vi "Set Header.vi"(7 "Replaced Existing (T)":bool=TRUE, 8 "error in (no error)":errorcluster, 9 "Value":string, 10 "Header":string, 11 "Response in":refnum<class "Response.lvclass">) -> (0 "error out":errorcluster, 1 "Replaced":bool, 3 "Response out":refnum<class "Response.lvclass">)   [LabVIEW 2020, in "HTTP Utils.lvlib" / "Response.lvclass"]
uses:
  Response.lvclass
  Response.lvclass/Response.ctl
  <vilib>/Utility/error.llb/Error Cluster From Error Code.vi
  <vilib>/ErrorRing/Error Ring.xnode
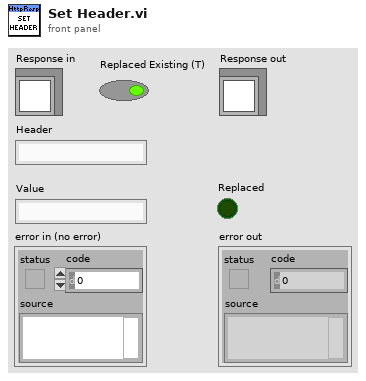
[diagram p1: front panel]
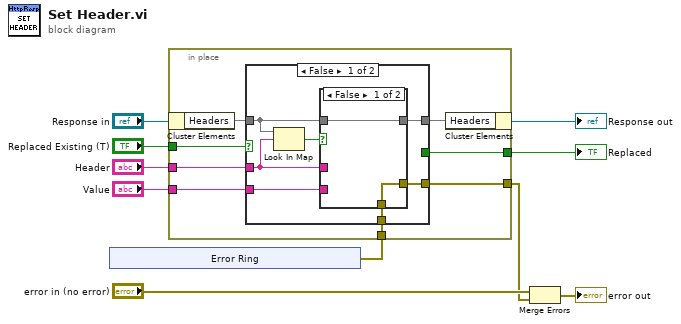
[diagram p0: block diagram]
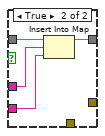
[diagram p2: hidden frame]
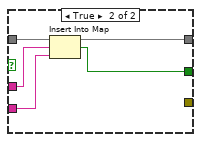
[diagram p3: hidden frame]
diagram:
  n1 = xnode "Error Ring"() -> ("error out"=w3:errorcluster)
  n2 = in-place {
    in-place-border: "Replaced Existing (T)" -> [w17]
    in-place-border: "Header" -> [w15]
    in-place-border: "Value" -> [w14]
    in-place-border: [w13] -> w5
    in-place-border: w3 -> [w12]
    in-place-border: [w11] -> w1
    n3 = in-place-cluster #1("Response in") -> ("Headers"=w18:map{string, string})
    n4 = case shown="False" w17 {
      tunnel: w18 -> [w25 w36]
      tunnel: [w21 w35] -> w16
      tunnel: w15 -> [w23 w34]
      tunnel: w14 -> [w22 w33]
      tunnel: [_ w32] -> w13
      tunnel: w12 -> [w20 _]
      tunnel: [w19 _] -> w11
      frame False {
        n5 = Look In Map(map=w25, key=w23) -> (key not found?=w24:bool)  [unwired: 1 in, 1 out]
        n6 = case shown="False" w24 {
          tunnel: w25 -> [w27 w31]
          tunnel: w23 -> [_ w30]
          tunnel: w22 -> [_ w29]
          tunnel: [w27 w28] -> w21
          tunnel: w20 -> [w26 _]
          tunnel: [w26 _] -> w19
          frame False {
          }
          frame True {
            n7 = Insert Into Map(map in=w31, key=w30, value=w29) -> (map out=w28:map{string, string})  [unwired: 2 out]
          }
        }
      }
      frame True {
        n8 = Insert Into Map(map in=w36, key=w34, value=w33) -> (map out=w35:map{string, string}, key already included?=w32:bool)  [unwired: 1 out]
      }
    }
    n9 = in-place-cluster #1("Headers"=w16) -> (→"Response out":refnum<class "Response.lvclass">)
  }
  "Replaced" <- w5
  n10 = Merge Errors("error in (no error)", w1) -> (→"error out":errorcluster)
